vi "PulseIntervalHistogram.vi"(9 "No of SI bins":dbl=50.0, 10 "Sampling interval":dbl, 11 "Binary array":bool[](array[boolean])) -> (2 "Pulse length histogram":T1(graph), 3 "Pulse period histogram":T1(graph))   [LabVIEW 2011]
uses:
  <vilib>/Analysis/NI_AALPro.lvlib
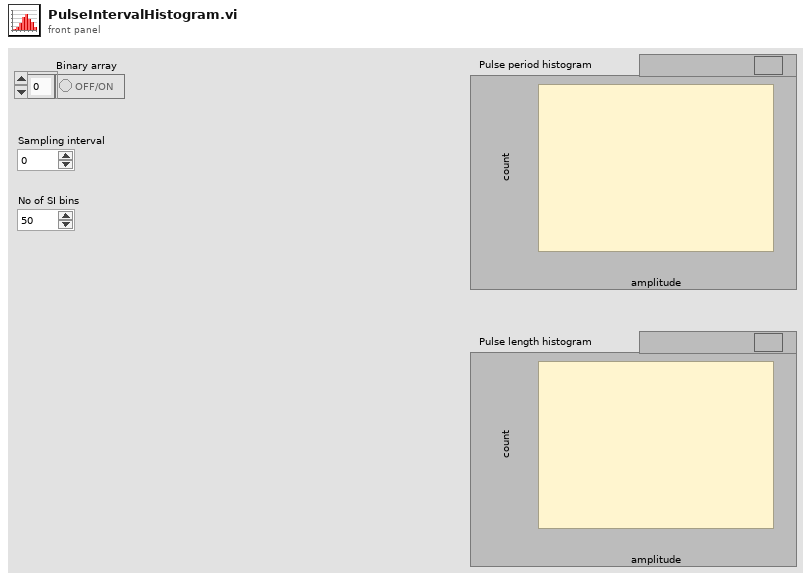
[diagram p1: front panel]
types:
  T1 = cluster{"X Values":dbl[], "Histogram: h(x)":i32[]}
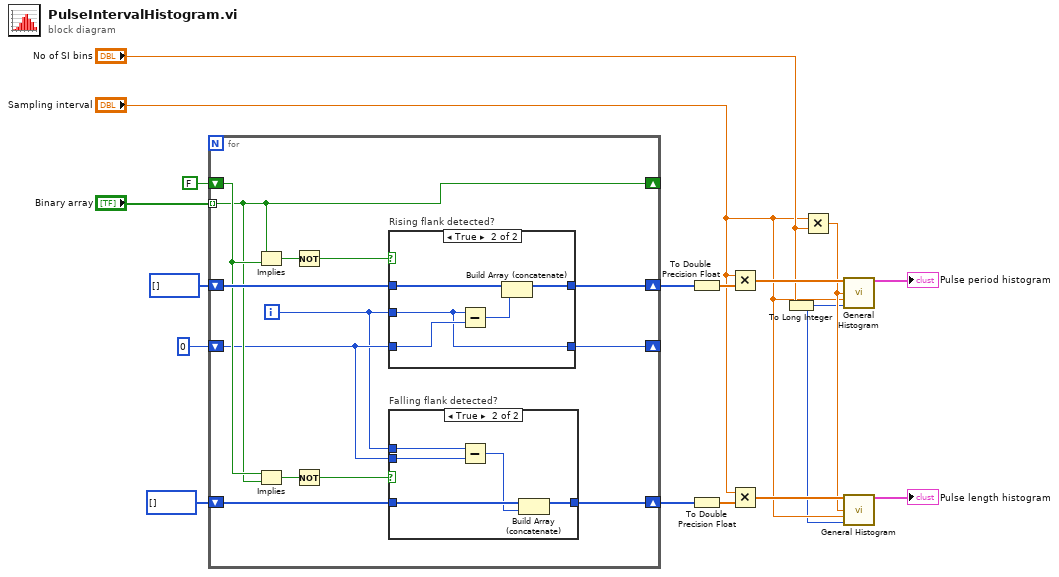
[diagram p0: block diagram]
diagram:
  n1 = for {
    tunnel: "Binary array" -> [w24] mode=indexing
    shift-right: [w24] -> _
    shift-left: FALSE -> [w25]
    shift-right: [w28] -> _
    shift-left: 0 -> [w20]
    shift-right: [w27] -> w13
    shift-left: i32[] [] -> [w26]
    shift-right: [w18] -> w6
    shift-left: i32[] [] -> [w21]
    i -> [w19]
    n2 = Implies(1:w25, 2:w24) -> (0:w30:bool)
    n3 = Implies(1:w24, 2:w25) -> (0:w23:bool)
    n4 = Not(x=w30) -> (.not. x?=w29:bool)
    n5 = Not(x=w23) -> (.not. x?=w22:bool)
    n6 = case "Rising flank detected?" shown="True" w29 {
      tunnel: w19 -> [_ w42]
      tunnel: [w38 w42] -> w28
      tunnel: w20 -> [w38 w43]
      tunnel: [w37 w40] -> w27
      tunnel: w26 -> [w37 w39]
      frame False {
      }
      frame True {
        n7 = Subtract(x=w42, y=w43) -> (x-y=w41:i32)
        n8 = Build Array (concatenate)(w39, w41) -> (w40:i32[])
      }
    }
    n9 = case "Falling flank detected?" shown="True" w22 {
      tunnel: w21 -> [w31 w34]
      tunnel: w20 -> [_ w35]
      tunnel: w19 -> [_ w36]
      tunnel: [w31 w32] -> w18
      frame False {
      }
      frame True {
        n10 = Subtract(x=w36, y=w35) -> (x-y=w33:i32)
        n11 = Build Array (concatenate)(w34, w33) -> (w32:i32[])
      }
    }
  }
  n12 = To Double Precision Float(number=w13) -> (double precision float=w12:dbl[])
  n13 = To Double Precision Float(number=w6) -> (double precision float=w7:dbl[])
  n14 = Multiply(x="Sampling interval", y=w12) -> (x*y=w11:dbl[])
  n15 = Multiply(x="Sampling interval", y=w7) -> (x*y=w5:dbl[])
  n16 = To Long Integer(number="No of SI bins") -> (32bit integer=w2:i32)
  n17 = Multiply(x="Sampling interval", y="No of SI bins") -> (x*y=w4:dbl)
  n18 = call <vilib>:"General Histogram.vi"("X"=w11, "max"=w4, "min"="Sampling interval", "# bins"=w2) -> ("Histogram Graph"=→"Pulse period histogram":T1)  [unwired: 7 in, 4 out]
  n19 = call <vilib>:"General Histogram.vi"("X"=w5, "max"=w4, "min"="Sampling interval", "# bins"=w2) -> ("Histogram Graph"=→"Pulse length histogram":T1)  [unwired: 7 in, 4 out]
